vi "Prepare file extension.vi"(4 "error in":errorcluster, 5 "input main cluster":T1) -> (0 "error out 2":errorcluster, 1 "output main cluster":T1)   [LabVIEW 2010]
uses:
  Main_cluster.ctl
  <vilib>/vision/Image Controls.llb/IMAQ Image.ctl
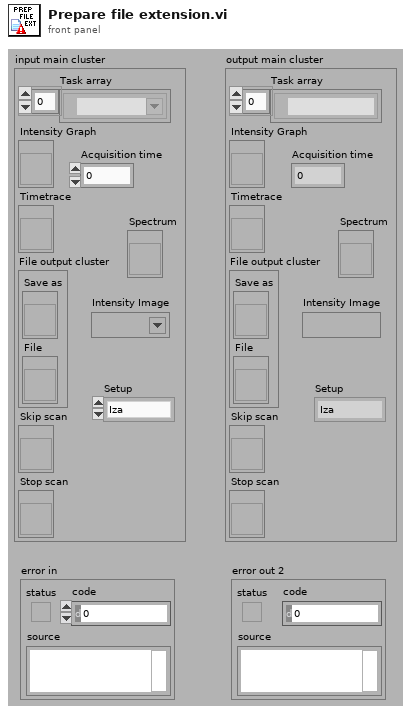
[diagram p1: front panel]
types:
  T1 = typedef "Main_cluster.ctl" = cluster{"Task array":refnum<k21>[], "Intensity Graph":refnum<vi>, "Timetrace":refnum<vi>, "File output cluster":cluster{"Save as":refnum<vi>, "File":refnum<vi>}, "Skip scan":refnum<vi>, "Stop scan":refnum<vi>, "Acquisition time":dbl, "Setup":enum16{"Iza", "Lukasz"}, "Spectrum":refnum<vi>, "Intensity Image":T2}
  T2 = typedef "IMAQ Image.ctl" = refnum<image>
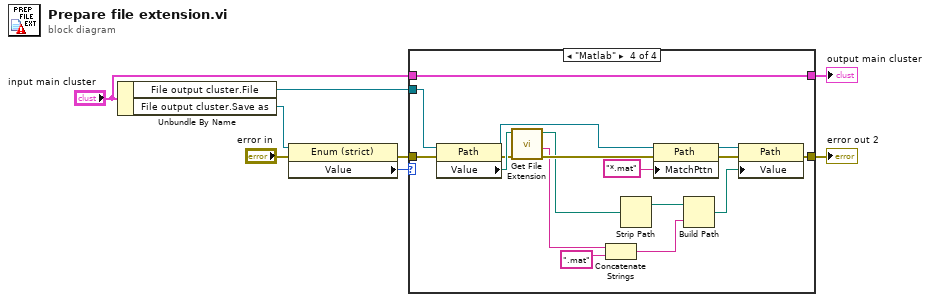
[diagram p0: block diagram]
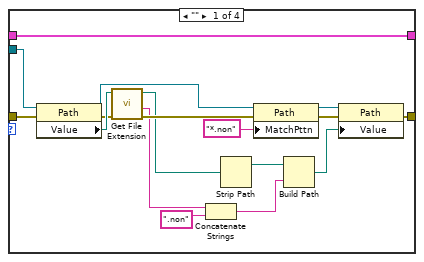
[diagram p2: hidden frame]
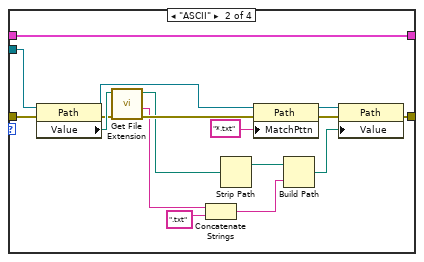
[diagram p3: hidden frame]
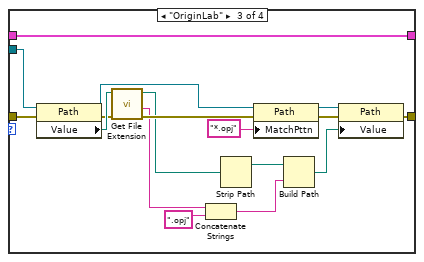
[diagram p4: hidden frame]
diagram:
  n1 = Unbundle By Name("input main cluster") -> ("File output cluster.File"=w1:refnum<vi>, "File output cluster.Save as"=w2:refnum<vi>)
  n2 = property class="Enum (strict)"(reference=w2, error in="error in") -> (error out=w3:errorcluster, "Value"=w7:enum16{"", "ASCII", "OriginLab", "Matlab"})  [unwired: 1 out]
  n3 = case shown="\"Matlab\"" w7 {
    tunnel: w3 -> [w13 w30 w47 w64]
    tunnel: [w10 w27 w44 w61] -> w5
    tunnel: "input main cluster" -> [w9 w26 w43 w60]
    tunnel: w1 -> [w18 w35 w52 w69]
    tunnel: [w9 w26 w43 w60] -> w8
    frame "" {
      n4 = property class="Path"(reference=w18, error in=w13) -> (reference out=w15:refnum<vi>, error out=w12:errorcluster, "Value"=w17:path)
      n5 = call <vilib>:"Get File Extension.vi"("error in (no error)"=w12, "file"=w17) -> ("error out"=w24:errorcluster, "filename without extension"=w23:string, "dup file"=w21:path)  [unwired: 6 in, 1 out]
      n6 = Concatenate Strings(w23, ".non" ("string")) -> (w19:string)
      n7 = Strip Path(path=w21) -> (stripped path=w20:path)  [unwired: 1 out]
      n8 = property on="Property Node" class="Path"(reference=w15, error in=w24, "MatchPttn"="*.non" ("Browse Options:Match Pattern")) -> (reference out=w14:refnum<vi>, error out=w11:errorcluster)
      n9 = Build Path(base path=w20, name or relative path=w19) -> (appended path=w16:path)
      n10 = property class="Path"(reference=w14, error in=w11, "Value"=w16) -> (error out=w10:errorcluster)  [unwired: 1 out]
    }
    frame "ASCII" {
      n11 = property class="Path"(reference=w35, error in=w30) -> (reference out=w32:refnum<vi>, error out=w29:errorcluster, "Value"=w34:path)
      n12 = call <vilib>:"Get File Extension.vi"("error in (no error)"=w29, "file"=w34) -> ("error out"=w41:errorcluster, "filename without extension"=w40:string, "dup file"=w38:path)  [unwired: 6 in, 1 out]
      n13 = Concatenate Strings(w40, ".txt" ("string")) -> (w36:string)
      n14 = Strip Path(path=w38) -> (stripped path=w37:path)  [unwired: 1 out]
      n15 = property on="Property Node" class="Path"(reference=w32, error in=w41, "MatchPttn"="*.txt" ("Browse Options:Match Pattern")) -> (reference out=w31:refnum<vi>, error out=w28:errorcluster)
      n16 = Build Path(base path=w37, name or relative path=w36) -> (appended path=w33:path)
      n17 = property class="Path"(reference=w31, error in=w28, "Value"=w33) -> (error out=w27:errorcluster)  [unwired: 1 out]
    }
    frame "OriginLab" {
      n18 = property class="Path"(reference=w52, error in=w47) -> (reference out=w49:refnum<vi>, error out=w46:errorcluster, "Value"=w51:path)
      n19 = call <vilib>:"Get File Extension.vi"("error in (no error)"=w46, "file"=w51) -> ("error out"=w58:errorcluster, "filename without extension"=w57:string, "dup file"=w55:path)  [unwired: 6 in, 1 out]
      n20 = Concatenate Strings(w57, ".opj" ("string")) -> (w53:string)
      n21 = Strip Path(path=w55) -> (stripped path=w54:path)  [unwired: 1 out]
      n22 = property on="Property Node" class="Path"(reference=w49, error in=w58, "MatchPttn"="*.opj" ("Browse Options:Match Pattern")) -> (reference out=w48:refnum<vi>, error out=w45:errorcluster)
      n23 = Build Path(base path=w54, name or relative path=w53) -> (appended path=w50:path)
      n24 = property class="Path"(reference=w48, error in=w45, "Value"=w50) -> (error out=w44:errorcluster)  [unwired: 1 out]
    }
    frame "Matlab" {
      n25 = property class="Path"(reference=w69, error in=w64) -> (reference out=w66:refnum<vi>, error out=w63:errorcluster, "Value"=w68:path)
      n26 = call <vilib>:"Get File Extension.vi"("error in (no error)"=w63, "file"=w68) -> ("error out"=w75:errorcluster, "filename without extension"=w74:string, "dup file"=w72:path)  [unwired: 6 in, 1 out]
      n27 = Concatenate Strings(w74, ".mat" ("string")) -> (w70:string)
      n28 = Strip Path(path=w72) -> (stripped path=w71:path)  [unwired: 1 out]
      n29 = property on="Property Node" class="Path"(reference=w66, error in=w75, "MatchPttn"="*.mat" ("Browse Options:Match Pattern")) -> (reference out=w65:refnum<vi>, error out=w62:errorcluster)
      n30 = Build Path(base path=w71, name or relative path=w70) -> (appended path=w67:path)
      n31 = property class="Path"(reference=w65, error in=w62, "Value"=w67) -> (error out=w61:errorcluster)  [unwired: 1 out]
    }
  }
  "output main cluster" <- w8
  "error out 2" <- w5
